vi "Errors Queue Ref.vi"(8 "error in (no error)":errorcluster) -> (0 "error out":errorcluster, 3 "queue out":refnum<queue>)   [LabVIEW 2019]
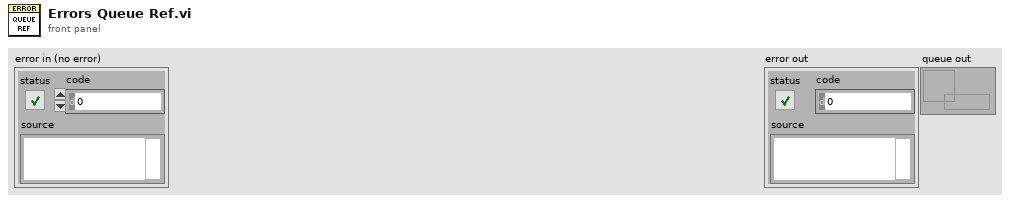
[diagram p1: front panel]
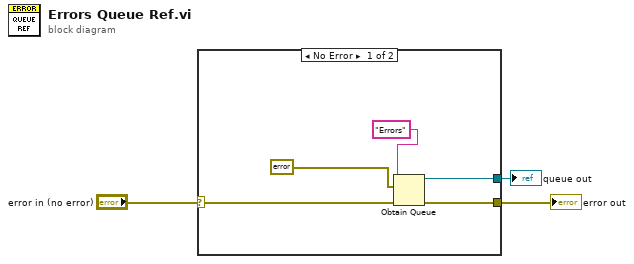
[diagram p0: block diagram]
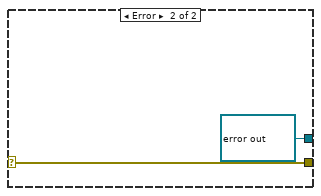
[diagram p2: hidden frame]
diagram:
  n1 = case shown="No Error" "error in (no error)" {
    selector: "error in (no error)" -> [w6 w10]
    tunnel: [w7 refnum<queue> refnum ("queue out")] -> w1
    tunnel: [w5 w10] -> w2
    frame No Error {
      n2 = Obtain Queue(name (unnamed)="Errors", element data type=errorcluster {"status"=FALSE, "code"=0, "source"=""} ("error out"), error in (no error)=w6) -> (queue out=w7:refnum<queue>, error out=w5:errorcluster)  [unwired: 2 in, 1 out]
    }
    frame Error {
    }
  }
  "error out" <- w2
  "queue out" <- w1
